vi "Control - Generic - Throttle Host.vi"() -> ()   [LabVIEW 2015, in "ECS-Host.lvlib"]
uses:
  ECS-Host.lvlib
  <vilib>/addons/Software Calibration Management/XControls/TBL2D.xctl
panel:
  out "ThrottlePsn_TblOut":sgl caption="[%Open]"
  in  "ThrottlePsn_Tbl":cluster{"X":sgl[], "Y":sgl[], "Z":sgl[][]}(xcontrol) caption="[bar|RPM|%Open]"
  in  "ThrottleCtrlMode":bool
  in  "ThrottlePsn_ManE":bool
  in  "ThrottlePsn_Man":sgl caption="[%Open]"
  out "ThrottlePsn_Des":sgl caption="[%Open]"
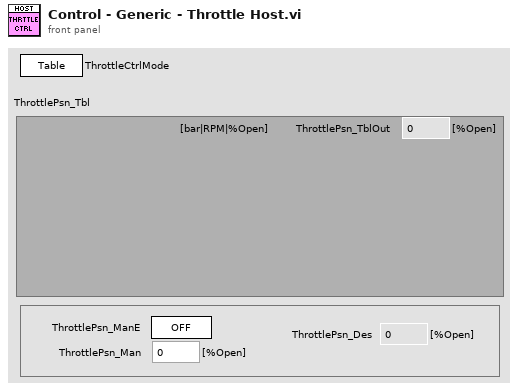
[diagram p1: front panel]
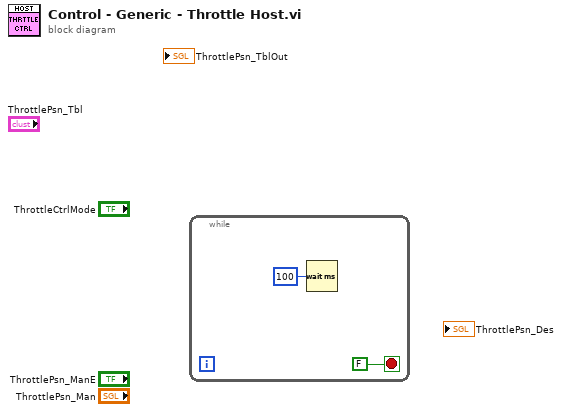
[diagram p0: block diagram]
diagram:
  n1 = while {
    stop <- FALSE stop-if-true
    n2 = Wait (ms)(milliseconds to wait=u32 100) -> ()  [unwired: 1 out]
  }
